vi "User Interface.vi"   [LabVIEW 2020, in "User Interface Utilities.lvlib"]
doc: "This template is for the Queued Message Handler design pattern.\n\nThe Event Handling Loop generates messages based on user interface actions.\n\nThe Message Handling Loop processes messages generated by the Event Handling Loop, or by other messages. The messages are string values, so new messages can be added easily to the Message Cases case structure in the Message Handling Loop. Each message cluster can also provide an optional value for Message Data, which is a variant that can be converted to whatever message-specific data is required."
uses:
  User Interface Utilities.lvlib
  Message Queue/Enqueue Message (Single).vi
  <vilib>/Utility/error.llb/Error Cluster From Error Code.vi
  <vilib>/ErrorRing/Error Ring.xnode
  Message Queue/Message Queue.lvlib
  Error Handler/Error Handler.lvlib
  User Event - Shutdown/User Event - Shutdown.lvlib
types:
  T1 = typedef "User Interface Utilities.lvlib/Message Queue.lvlib/All Message Queues.ctl" = cluster{"UI":refnum<queue>}
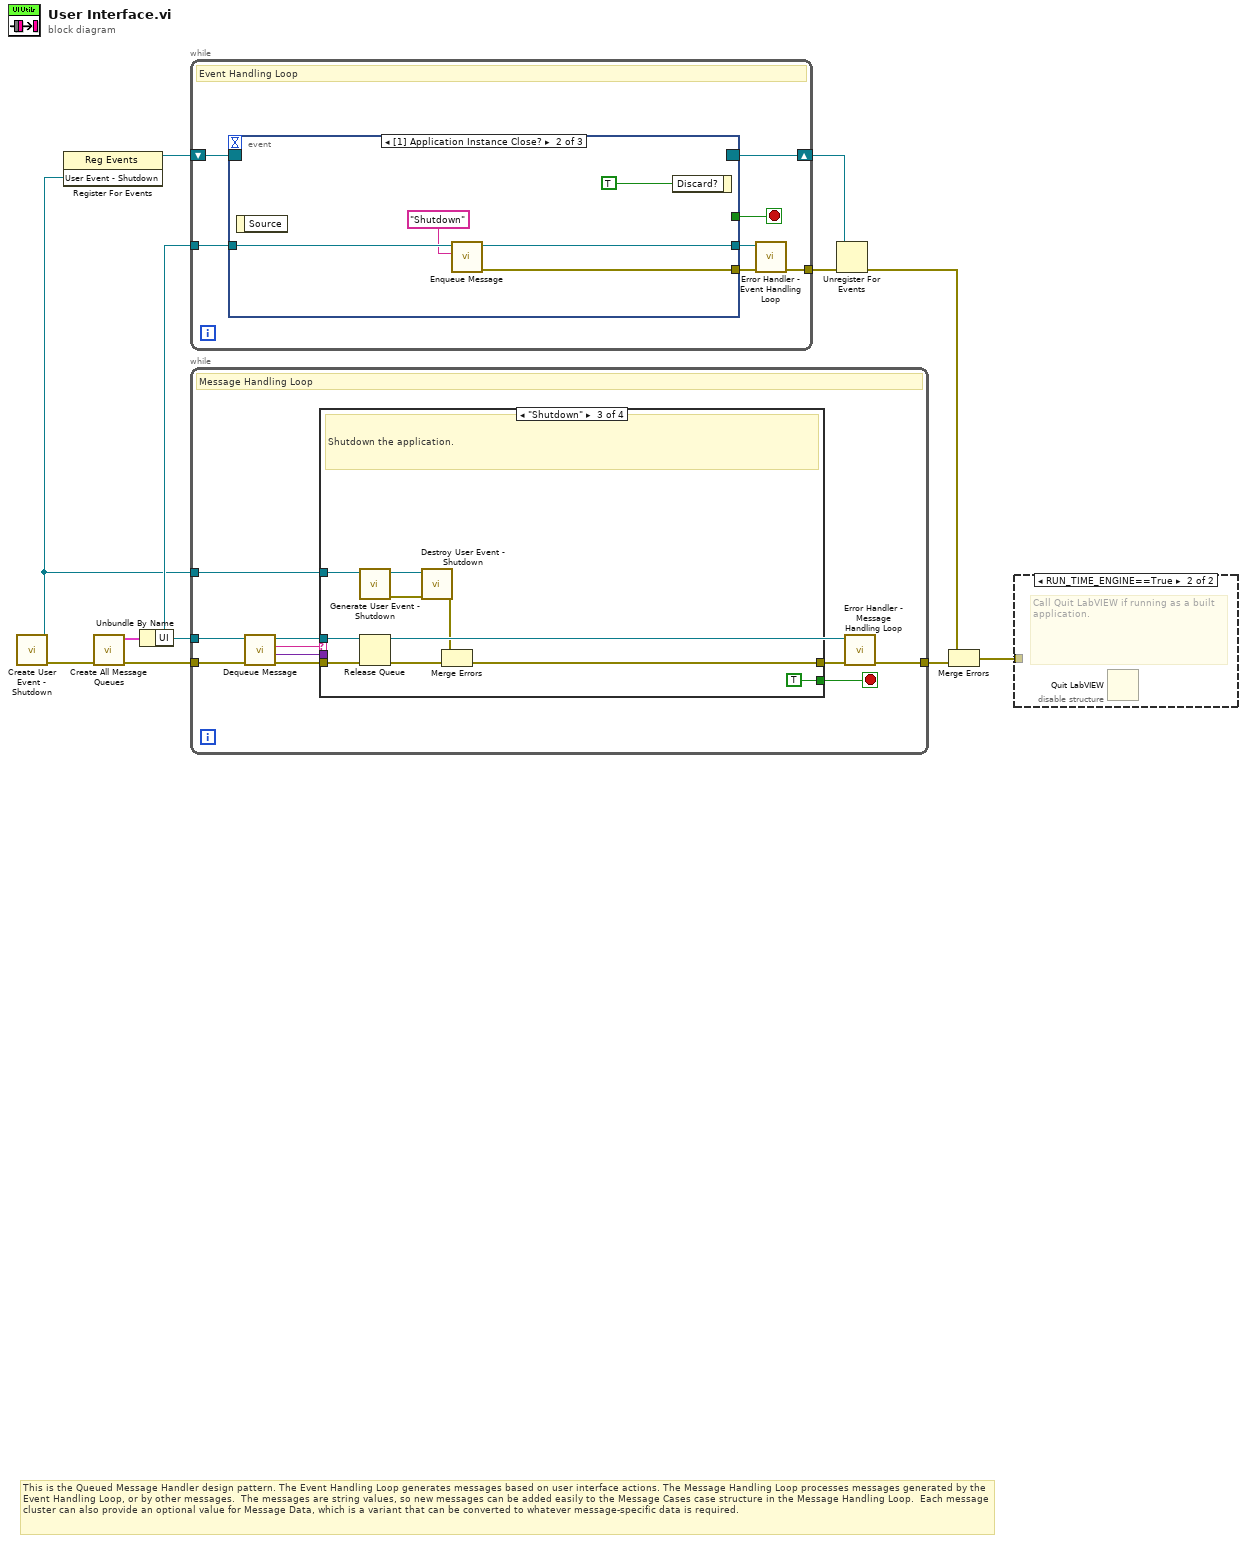
[diagram p0: block diagram]
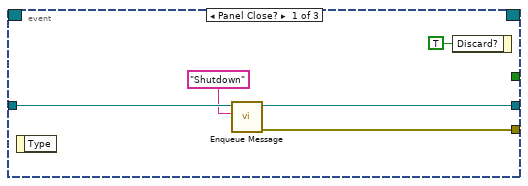
[diagram p3: hidden frame]
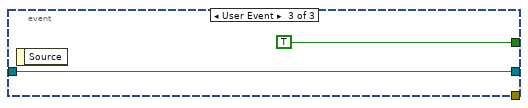
[diagram p4: hidden frame]
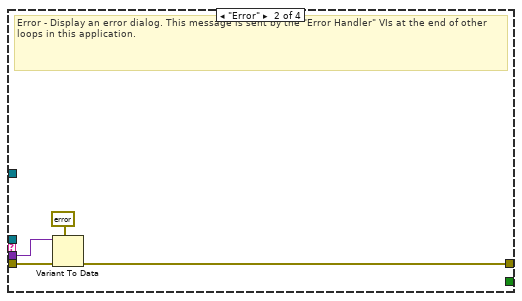
[diagram p6: hidden frame]
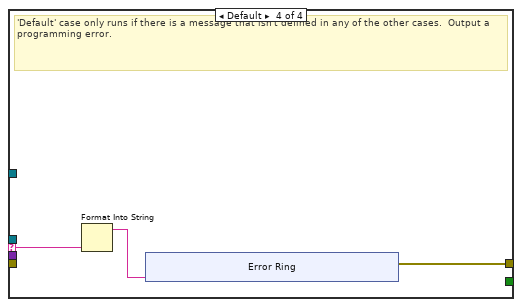
[diagram p7: hidden frame]
diagram:
  # "This is the Queued Message Handler design pattern. The Event Handling Loop generates messages based on user interface actions. The Message Handling Loop processes messages generated by the Event Handling Loop, or by other messages.  The messages are string values, so new messages can be added easily to the Message Cases case structure in the Message Handling Loop.  Each message cluster can also provide an optional value for Message Data, which is a variant that can be converted to whatever message-specific data is required."
  n1 = call "Create User Event - Shutdown.vi"() -> ("error out"=w7:errorcluster, "User Event - Shutdown"=w3:refnum<user-event>)  [unwired: 10 in]
  n2 = register-events(w3) -> (reference out=w2:refnum<event-registration>)  [unwired: 2 in, 1 out]
  n3 = call "Create All Message Queues.vi"("error in (no error)"=w7) -> ("error out"=w10:errorcluster, "Message Queues out"=w9:T1)  [unwired: 9 in]
  n4 = Unbundle By Name(w9) -> ("UI"=w8:refnum<queue>)
  n5 = while {
    tunnel: w8 -> [w18]
    shift-right: [w16] -> w6
    shift-left: w2 -> [w17]
    tunnel: [w12] -> w5
    stop <- w14 stop-if-true
    # "Event Handling Loop"
    n6 = event shown="[1] Application Instance Close?" {
      selector: w17 -> [_ _ _]
      dyn-events: [_ _ _] -> w16
      timeout: _ -> [_ _ _]
      tunnel: [_ _ TRUE ("Discard?")] -> w14
      tunnel: w18 -> [w22 w28 w30]
      tunnel: [w21 w27 _] -> w15
      tunnel: [w20 w26 w30] -> w13
      event Panel Close? {
        n7 = event-data() -> ()  [unwired: 1 in, 1 out]
        n8 = call-poly "Enqueue Message.vi"("Action"="Shutdown", "Message Queue"=w22) -> ("error out"=w21:errorcluster, "dup Message Queue"=w20:refnum<queue>)  [unwired: 8 in]
        n9 = event-data("Discard?"=TRUE) -> ()  [unwired: 1 in, 1 out]
      }
      event Application Instance Close? {
        n10 = event-data() -> ()  [unwired: 1 in, 1 out]
        n11 = call-poly "Enqueue Message.vi"("Action"="Shutdown", "Message Queue"=w28) -> ("error out"=w27:errorcluster, "dup Message Queue"=w26:refnum<queue>)  [unwired: 8 in]
        n12 = event-data("Discard?"=TRUE) -> ()  [unwired: 1 in, 1 out]
      }
      event User Event {
        n13 = event-data() -> ()  [unwired: 1 in, 1 out]
      }
    }
    n14 = call "Error Handler - Event Handling Loop.vi"("error in (no error)"=w15, "Message Queue"=w13) -> ("dup error in"=w12:errorcluster)  [unwired: 8 in, 1 out]
  }
  n15 = while {
    tunnel: w8 -> [w34]
    tunnel: w3 -> [w39]
    tunnel: w10 -> [w38]
    tunnel: [w33] -> w4
    stop <- w40 stop-if-true
    # "Message Handling Loop"
    n16 = call "Dequeue Message.vi"("error in (no error)"=w38, "Message Queue"=w34) -> ("error out"=w37:errorcluster, "Message Data"=w35:variant, "Action"=w36:string, "dup Message Queue"=w31:refnum<queue>)  [unwired: 6 in]
    n17 = case "Message Cases" shown="\"Shutdown\"" w36 {
      selector: w36 -> [_ _ _ w56]
      tunnel: w31 -> [_ _ w54 _]
      tunnel: w37 -> [w41 w45 w50 _]
      tunnel: [w41 w43 w51 w57] -> w32
      tunnel: [_ _ TRUE _] -> w40
      tunnel: w35 -> [_ w44 _ _]
      tunnel: w39 -> [_ _ w48 _]
      frame "Initialize" {
        # "Initialize - All initialization work should take place in this message, since other loops can potentially enqueue messages that execute immediately after this one."
      }
      frame "Error" {
        # "Error - Display an error dialog. This message is sent by the \"Error Handler\" VIs at the end of other loops in this application."
        n18 = Variant To Data(error in=w45, type=errorcluster {"status"=FALSE, "code"=0, "source"=""} ("error in (no error)"), Variant=w44) -> (error out=w43:errorcluster)  [unwired: 1 out]
      }
      frame "Shutdown" {
        # "Shutdown the application."
        n19 = call "Generate User Event - Shutdown.vi"("User Event - Shutdown"=w48) -> ("error out"=w49:errorcluster, "User Event - Shutdown out"=w46:refnum<user-event>)  [unwired: 9 in]
        n20 = Release Queue(queue=w54, error in (no error)=w50) -> (error out=w52:errorcluster)  [unwired: 1 in, 2 out]
        n21 = call "Destroy User Event - Shutdown.vi"("error in (no error)"=w49, "User Event - Shutdown"=w46) -> ("error out"=w47:errorcluster)  [unwired: 9 in]
        n22 = Merge Errors(w47, w52) -> (w51:errorcluster)
      }
      frame Default {
        # "'Default' case only runs if there is a message that isn't defined in any of the other cases.  Output a programming error."
        n23 = Format Into String(w56) -> (resulting string=w55:string)  [unwired: 3 in, 1 out]
        n24 = xnode "Error Ring"("parameter 0"=w55) -> ("error out"=w57:errorcluster)
      }
    }
    n25 = call "Error Handler - Message Handling Loop.vi"("error in (no error)"=w32, "Message Queue"=w31) -> ("dup error in"=w33:errorcluster)  [unwired: 8 in, 1 out]
  }
  n26 = Unregister For Events(event registration refnum=w6, error in=w5) -> (error out=w11:errorcluster)
  n27 = Merge Errors(w11, w4) -> (w1:errorcluster)
  n28 = disable-structure shown="RUN_TIME_ENGINE==True" {
    disable-tunnel: w1 -> [_ _]
    frame condition #0 (active) {
    }
    frame condition #1 {
      # "Call Quit LabVIEW if running as a built application."
      n29 = Quit LabVIEW() -> ()  [unwired: 1 in]
    }
  }
